vi "Write to Observer.vi"(8 "error in":errorcluster, 11 "tCRD in":refnum<class "Open Path CRD.lvclass">) -> (0 "error out":errorcluster, 3 "tCRD out":refnum<class "Open Path CRD.lvclass">)   [LabVIEW 2015, in "Open Path CRD.lvclass"]
uses:
  Open Path CRD.lvclass
  Reusable/File IO/Class/File Observer.lvclass
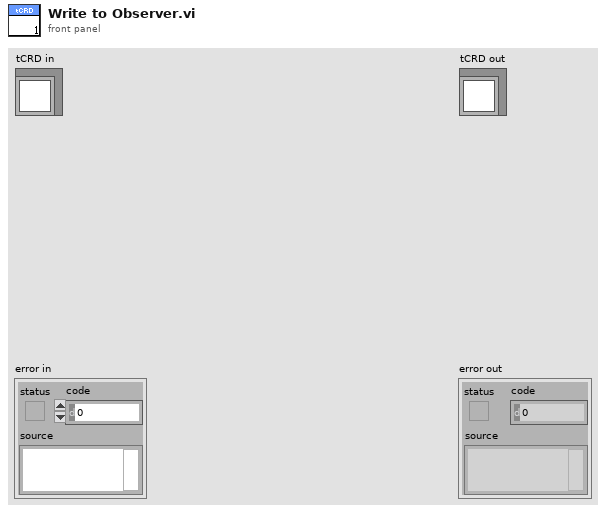
[diagram p1: front panel]
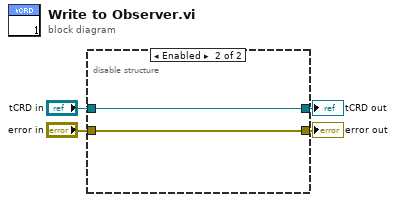
[diagram p0: block diagram]
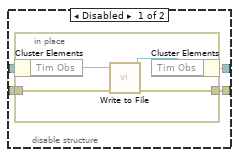
[diagram p2: hidden frame]
diagram:
  n1 = disable-structure shown="Enabled" {
    disable-tunnel: "error in" -> [w8 w13]
    disable-tunnel: [w7 w13] -> w3
    disable-tunnel: "tCRD in" -> [w6 w14]
    disable-tunnel: [w5 w14] -> w1
    frame Disabled {
      n2 = in-place {
        in-place-border: w8 -> [w10]
        in-place-border: [w9] -> w7
        n3 = in-place-cluster #1(w6) -> ("Tim Obs"=w12:refnum<class "Tim File Observer.lvclass">)
        n4 = call "Write to File.vi"("error in"=w10, "File Obs in"=w12) -> ("error out"=w9:errorcluster, "File Obs out"=w11:refnum<class "Tim File Observer.lvclass">)  [unwired: 8 in]
        n5 = in-place-cluster #1("Tim Obs"=w11) -> (w5:refnum<class "Open Path CRD.lvclass">)
      }
    }
    frame Enabled {
    }
  }
  "error out" <- w3
  "tCRD out" <- w1
